vi "Periodic Tasks.vi"(8 "error in":errorcluster) -> ()   [LabVIEW 2012]
doc: "This VI runs in parallel to other tasks. It can contain as many user-defined periodic loops as you need. These can carry out PID or other sorts of timed response."
uses:
  <vilib>/Rock Robotics/SystemInterfaces/Utilities/FPGA_UtilitiesLED Source.ctl
  <vilib>/Rock Robotics/SystemInterfaces/Utilities/FPGA_UtilitiesLED State.ctl
  <vilib>/Rock Robotics/WPI/Solenoid/WPI_SolenoidValue.ctl
  Robot Global Data.vi
  <vilib>/Rock Robotics/WPI/Solenoid/WPI_SolenoidSetEnum.vi
  <vilib>/Rock Robotics/WPI/Compressor/WPI_CompressorGetSetRefNum.vi
panel:
  out "RawPot1":dbl
  out "RawGyro":dbl
  out "Pot1":dbl
  out "Gyro1":dbl
  out "PickupErrort":errorcluster
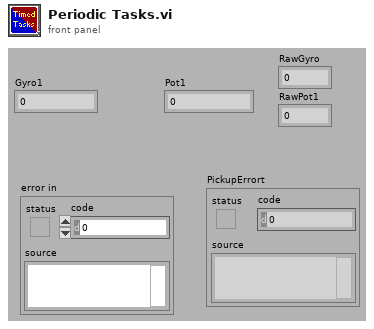
[diagram p1: front panel]
types:
  T1 = typedef "FPGA_UtilitiesLED State.ctl" = enum16{"Off", "On", "Toggle"}
  T2 = typedef "FPGA_UtilitiesLED Source.ctl" = enum16{"User LED", "FPGA LED"}
  T3 = typedef "WPI_MotorControlDeviceRef.ctl" = cluster{"DeviceStatus":errorcluster, "Type":enum16{"PWM", "CAN"}, "PWM":cluster{"Digital Module":T4, "PWM Channel":T5, "DeadBand":T6}, "CAN":cluster{"Device Number":u8, "Control Mode":T7, "Semaphore":T8, "Max Vout":dbl}, "Invert":bool, "TransformRef":T9, "InvTransformRef":T9}
  T4 = typedef "FPGA_TypedefDigitalModule.ctl" = enum16{"Digital Module 1", "Digital Module 2"}
  T5 = typedef "FPGA_DIOPWMChannel.ctl" = enum8{"PWM 1", "PWM 2", "PWM 3", "PWM 4", "PWM 5", "PWM 6", "PWM 7", "PWM 8", "PWM 9", "PWM 10", "Invalid"}
  T6 = typedef "WPI_PWMDeadband.ctl" = cluster{"Name":string, "maxPositivePwm":i32, "minPositivePwm":i32, "centerPwm":i32, "maxNegativePwm":i32, "minNegativePwm":i32, "angularRange":u16}
  T7 = typedef "WPI_CANJaguar_ControlMode.ctl" = enum8{"Percent VBus", "Current", "Speed", "Position", "Voltage"}
  T8 = typedef "Semaphore RefNum" = refnum<k1>
  T9 = typedef "WPI_PWMTransform_ConPane.ctl" = refnum<vi>
  T10 = typedef "WPI_SolenoidDevRef.ctl" = cluster{"DevStatus":errorcluster, "Solenoid Module":T11, "Forward Solenoid Channel":T12, "Reverse Solenoid Channel":T12}
  T11 = typedef "FPGA_TypedefSolenoidModule.ctl" = enum16{"Solenoid Module 1", "Solenoid Module 2"}
  T12 = typedef "WPI_SolenoidChannel.ctl" = enum8{"Solenoid 1", "Solenoid 2", "Solenoid 3", "Solenoid 4", "Solenoid 5", "Solenoid 6", "Solenoid 7", "Solenoid 8", "Invalid"}
  T13 = typedef "WPI_CompressorDevRef.ctl" = cluster{"DevStatus":errorcluster, "DigitalInputDevRef":T14, "RelayDevRef":T16}
  T14 = typedef "WPI_DigitalInputDevRef.ctl" = cluster{"DevStatus":errorcluster, "DIO Channel":T15, "Digital Module":T4}
  T15 = typedef "FPGA_DIOChannel.ctl" = enum8{"DIO 1", "DIO 2", "DIO 3", "DIO 4", "DIO 5", "DIO 6", "DIO 7", "DIO 8", "DIO 9", "DIO 10", "DIO 11", "DIO 12", "DIO 13", "DIO 14", "Invalid"}
  T16 = typedef "WPI_RelayDevRef.ctl" = cluster{"DevStatus":errorcluster, "Relay Channel":T17, "Digital Module":T4, "Relay Direction":T18}
  T17 = typedef "FPGA_DIORelayChannel.ctl" = enum8{"Relay 1", "Relay 2", "Relay 3", "Relay 4", "Relay 5", "Relay 6", "Relay 7", "Relay 8", "Invalid"}
  T18 = typedef "WPI_RelayDirection.ctl" = enum16{"Both directions", "Forward only", "Reverse only"}
  T19 = typedef "WPI_GyroDevRef.ctl" = cluster{"DevStatus":errorcluster, "Analog Module":T20, "Analog Channel":T21, "Offset":dbl, "Gain (VoltsPerDegree/Second)":dbl}
  T20 = typedef "FPGA_TypedefAnalogModule.ctl" = enum16{"Analog Module 1", "Analog Module 2"}
  T21 = typedef "FPGA_AIChannel.ctl" = enum8{"AI 1", "AI 2", "AI 3", "AI 4", "AI 5", "AI 6", "AI 7", "AI 8", "Invalid"}
  T22 = typedef "WPI_AnalogChannelDevRef.ctl" = cluster{"DevStatus":errorcluster, "Analog Module":T20, "Analog Channel":T21}
  T23 = enum16{"Reset", "Ready", "Down", "Capture", "Lift", "Swing", "Release"}
  T24 = typedef "WPI_SolenoidValue.ctl" = enum16{"Off", "On", "Forward", "Reverse"}
  T25 = cluster{"PizzaLow":dbl, "PizzaMid":dbl, "PizzaTop":dbl}
  T26 = cluster{"Shoot":bool, "Enable_Targeting":bool, "Shooter":dbl, "LeadScrew":dbl, "Feed":bool, "Pickup":bool}
  T27 = cluster{"Frisbee_Catch":bool, "Shooter_Ready":bool, "LeadScrewEnd":bool}
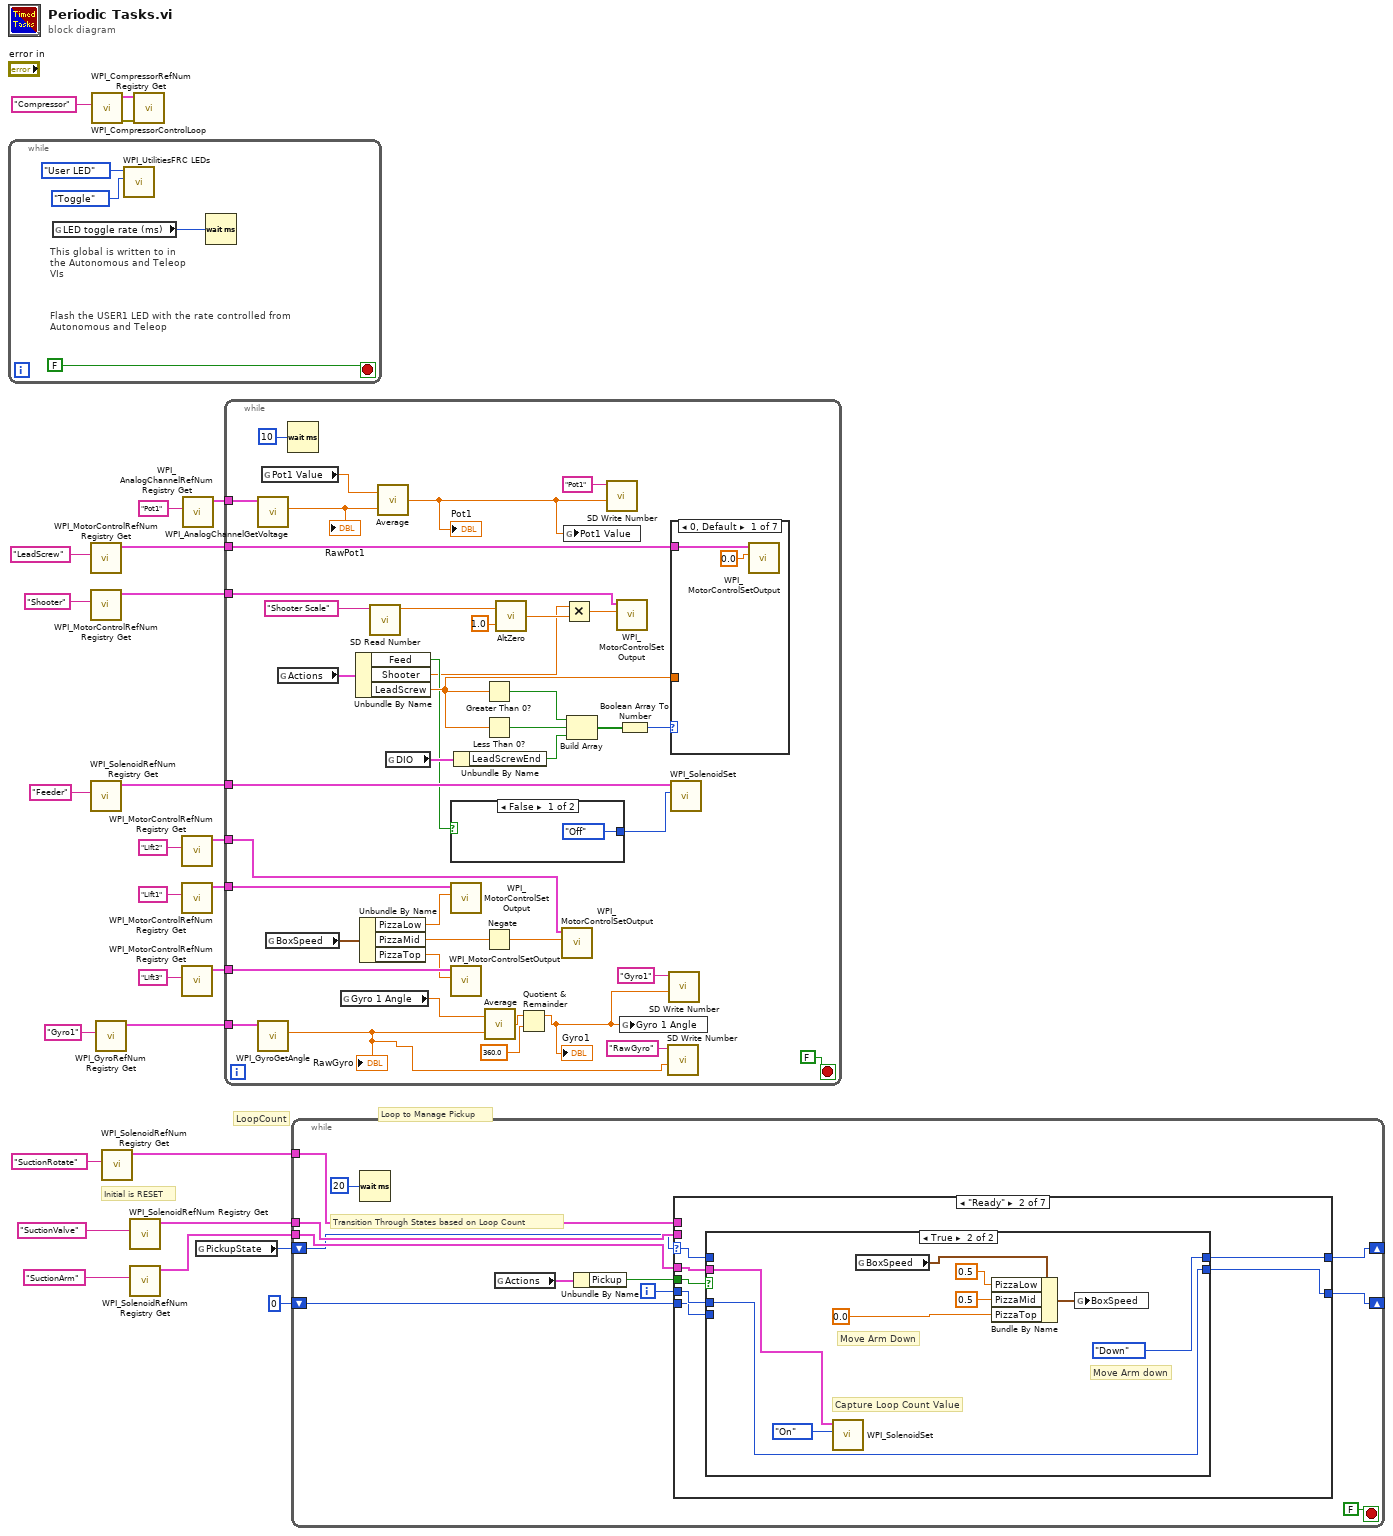
[diagram p0: block diagram]
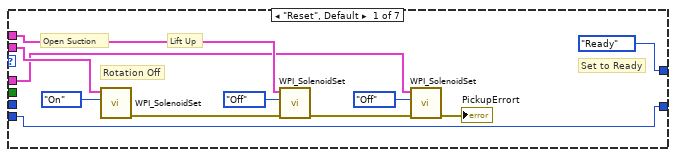
[diagram p2: hidden frame]
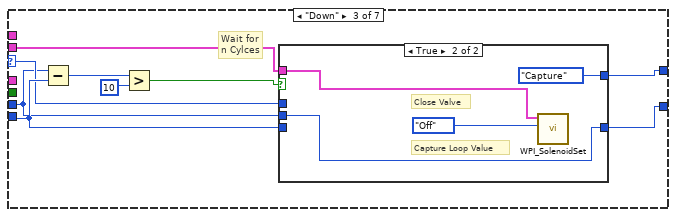
[diagram p4: hidden frame]
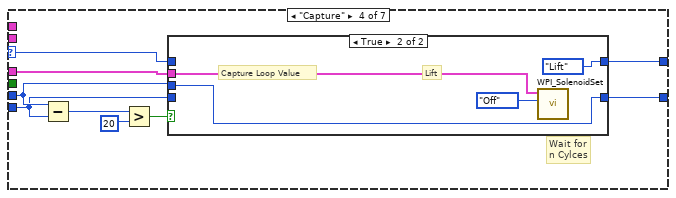
[diagram p6: hidden frame]
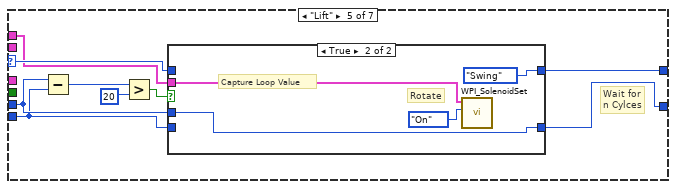
[diagram p8: hidden frame]
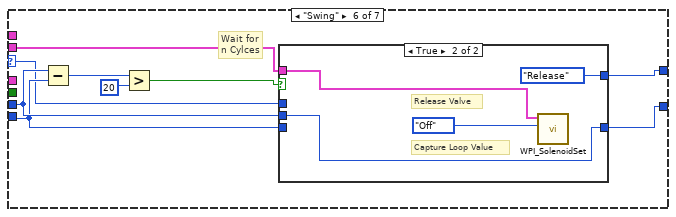
[diagram p10: hidden frame]
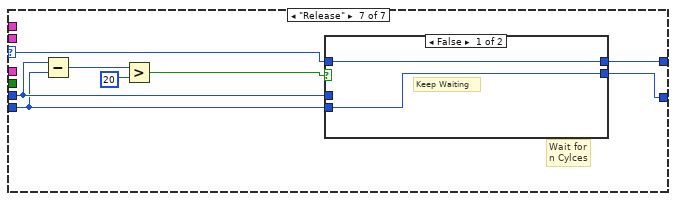
[diagram p12: hidden frame]
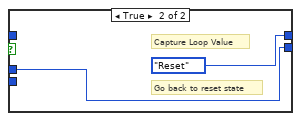
[diagram p13: hidden frame]
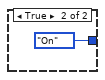
[diagram p14: hidden frame]
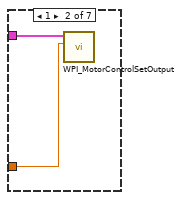
[diagram p15: hidden frame]
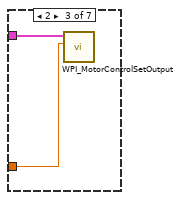
[diagram p16: hidden frame]
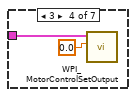
[diagram p17: hidden frame]
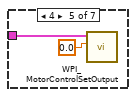
[diagram p18: hidden frame]
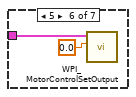
[diagram p19: hidden frame]
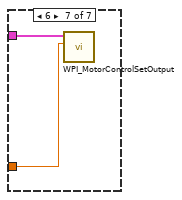
[diagram p20: hidden frame]
diagram:
  # "Initial is RESET"
  # "LoopCount"
  # "Loop to Manage Pickup"
  n1 = while {
    stop <- FALSE stop-if-true
    # "This global is written to in the Autonomous and Teleop VIs"
    # "Flash the USER1 LED with the rate controlled from Autonomous and Teleop"
    n2 = global read "Robot Global Data.vi" "LED toggle rate (ms)"() -> (w28:u32)
    n3 = call <vilib>:"WPI_UtilitiesFRC LEDs.vi"("State"=FPGA_UtilitiesLED_State."Toggle", "LED Type"=FPGA_UtilitiesLED_Source."User LED") -> ()  [unwired: 1 in, 9 out]
    n4 = Wait (ms)(milliseconds to wait=w28) -> ()  [unwired: 1 out]
  }
  n5 = call <vilib>:"WPI_MotorControlRefNum Registry Get.vi"("refnum name"="LeadScrew") -> ("MotorControlDevRef"=w23:T3)  [unwired: 9 in, 1 out]
  n6 = call <vilib>:"WPI_MotorControlRefNum Registry Get.vi"("refnum name"="Shooter") -> ("MotorControlDevRef"=w21:T3)  [unwired: 9 in, 1 out]
  n7 = call <vilib>:"WPI_SolenoidRefNum Registry Get.vi"("refnum name"="Feeder") -> ("SolenoidDevRef"=w20:T10)  [unwired: 9 in, 1 out]
  n8 = call <vilib>:"WPI_CompressorRefNum Registry Get.vi"("refnum name"="Compressor") -> ("error out"=w25:errorcluster, "CompressorDevRef"=w27:T13)  [unwired: 9 in]
  n9 = call <vilib>:"WPI_GyroRefNum Registry Get.vi"("refnum name"="Gyro1") -> ("GyroDevRef"=w3:T19)  [unwired: 9 in, 1 out]
  n10 = call <vilib>:"WPI_SolenoidRefNum Registry Get.vi"("refnum name"="SuctionRotate") -> ("SolenoidDevRef"=w13:T10)  [unwired: 9 in, 1 out]
  n11 = call <vilib>:"WPI_SolenoidRefNum Registry Get.vi"("refnum name"="SuctionValve") -> ("SolenoidDevRef"=w15:T10)  [unwired: 9 in, 1 out]
  n12 = call <vilib>:"WPI_SolenoidRefNum Registry Get.vi"("refnum name"="SuctionArm") -> ("SolenoidDevRef"=w14:T10)  [unwired: 9 in, 1 out]
  n13 = call <vilib>:"WPI_CompressorControlLoop.vi"("error in (no error)"=w25, "CompressorDevRef"=w27) -> ()  [unwired: 10 in]
  n14 = call <vilib>:"WPI_MotorControlRefNum Registry Get.vi"("refnum name"="Lift2") -> ("MotorControlDevRef"=w5:T3)  [unwired: 9 in, 1 out]
  n15 = call <vilib>:"WPI_MotorControlRefNum Registry Get.vi"("refnum name"="Lift1") -> ("MotorControlDevRef"=w7:T3)  [unwired: 9 in, 1 out]
  n16 = call <vilib>:"WPI_MotorControlRefNum Registry Get.vi"("refnum name"="Lift3") -> ("MotorControlDevRef"=w6:T3)  [unwired: 9 in, 1 out]
  n17 = call <vilib>:"WPI_AnalogChannelRefNum Registry Get.vi"("refnum name"="Pot1") -> ("AIDeviceRef"=w1:T22)  [unwired: 9 in, 1 out]
  n18 = global read "Robot Global Data.vi" "PickupState"() -> (w12:T23)
  n19 = while {
    tunnel: w23 -> [w66]
    tunnel: w21 -> [w65]
    tunnel: w20 -> [w61]
    tunnel: w7 -> [w57]
    tunnel: w6 -> [w56]
    tunnel: w5 -> [w55]
    tunnel: w3 -> [w50]
    tunnel: w1 -> [w42]
    stop <- FALSE stop-if-true
    n20 = call <vilib>:"WPI_AnalogChannelGetVoltage.vi"("AIDeviceRef"=w42) -> ("Voltage"=w39:dbl)  [unwired: 8 in, 2 out]
    "RawPot1" <- w39
    n21 = call <vilib>:"WPI_GyroGetAngle.vi"("GyroDevRef"=w50) -> ("Angle"=w33:dbl)  [unwired: 7 in, 3 out]
    "RawGyro" <- w33
    n22 = global read "Robot Global Data.vi" "Pot1 Value"() -> (w40:dbl)
    n23 = global read "Robot Global Data.vi" "BoxSpeed"() -> (w58:T25)
    n24 = global read "Robot Global Data.vi" "Actions"() -> (w64:T26)
    n25 = Wait (ms)(milliseconds to wait=u32 10) -> ()  [unwired: 1 out]
    n26 = global read "Robot Global Data.vi" "Gyro 1 Angle"() -> (w41:dbl)
    n27 = Unbundle By Name(w64) -> ("Feed"=w59:bool, "Shooter"=w44:dbl, "LeadScrew"=w60:dbl)
    n28 = Unbundle By Name(w58) -> ("PizzaLow"=w54:dbl, "PizzaMid"=w52:dbl, "PizzaTop"=w51:dbl)
    n29 = call <vilib>:"SD Read Number.vi"("Name"="Shooter Scale") -> ("Numeric"=w46:dbl)  [unwired: 8 in, 2 out]
    n30 = call "Average.vi"("z"=w39, "x"=w40) -> ("y"=w38:dbl)
    "Pot1" <- w38
    n31 = global read "Robot Global Data.vi" "DIO"() -> (w63:T27)
    n32 = case shown="False" w59 {
      tunnel: [WPI_SolenoidValue."Off" ("Value") WPI_SolenoidValue."On" ("Value")] -> w62
      frame False {
      }
      frame True {
      }
    }
    n33 = call <vilib>:"WPI_MotorControlSetOutput.vi"("Output"=w54, "MotorControlDevRef"=w57) -> ()  [unwired: 7 in, 3 out]
    n34 = call <vilib>:"WPI_MotorControlSetOutput.vi"("Output"=w51, "MotorControlDevRef"=w56) -> ()  [unwired: 7 in, 3 out]
    n35 = Unbundle By Name(w63) -> ("LeadScrewEnd"=w67:bool)
    n36 = Greater Than 0?(x=w60) -> (x > 0?=w70:bool)
    n37 = Less Than 0?(x=w60) -> (x < 0?=w71:bool)
    n38 = Negate(x=w52) -> (-x=w53:dbl)
    n39 = call "Average.vi"("z"=w33, "x"=w41) -> ("y"=w36:dbl)
    n40 = call "AltZero.vi"("z"=1.0, "x"=w46) -> ("y"=w47:dbl)
    n41 = Quotient & Remainder(x=w36, y=360.0) -> (x-y*floor(x/y)=w35:dbl)  [unwired: 1 out]
    "Gyro1" <- w35
    n42 = call <vilib>:"WPI_MotorControlSetOutput.vi"("Output"=w53, "MotorControlDevRef"=w55) -> ()  [unwired: 7 in, 3 out]
    n43 = global write "Robot Global Data.vi" "Pot1 Value"(w38) -> ()
    n44 = Multiply(x=w44, y=w47) -> (x*y=w43:dbl)
    n45 = Build Array(w70, w71, w67) -> (w69:bool[])
    n46 = call <vilib>:"SD Write Number.vi"("Numeric"=w38, "Name"="Pot1") -> ()  [unwired: 8 in, 2 out]
    n47 = call <vilib>:"WPI_MotorControlSetOutput.vi"("Output"=w43, "MotorControlDevRef"=w65) -> ()  [unwired: 7 in, 3 out]
    n48 = Boolean Array To Number(Boolean array=w69) -> (number=w68:u32)
    n49 = global write "Robot Global Data.vi" "Gyro 1 Angle"(w35) -> ()
    n50 = call <vilib>:"SD Write Number.vi"("Numeric"=w33, "Name"="RawGyro") -> ()  [unwired: 8 in, 2 out]
    n51 = call <vilib>:"SD Write Number.vi"("Numeric"=w35, "Name"="Gyro1") -> ()  [unwired: 8 in, 2 out]
    n52 = case shown="0, Default" w68 {
      tunnel: w60 -> [_ w79 w81 _ _ _ w88]
      tunnel: w66 -> [w76 w78 w80 w83 w85 w87 w89]
      frame 0, Default {
        n53 = call <vilib>:"WPI_MotorControlSetOutput.vi"("Output"=0.0, "MotorControlDevRef"=w76) -> ()  [unwired: 7 in, 3 out]
      }
      frame 1 {
        n54 = call <vilib>:"WPI_MotorControlSetOutput.vi"("Output"=w79, "MotorControlDevRef"=w78) -> ()  [unwired: 7 in, 3 out]
      }
      frame 2 {
        n55 = call <vilib>:"WPI_MotorControlSetOutput.vi"("Output"=w81, "MotorControlDevRef"=w80) -> ()  [unwired: 7 in, 3 out]
      }
      frame 3 {
        n56 = call <vilib>:"WPI_MotorControlSetOutput.vi"("Output"=0.0, "MotorControlDevRef"=w83) -> ()  [unwired: 7 in, 3 out]
      }
      frame 4 {
        n57 = call <vilib>:"WPI_MotorControlSetOutput.vi"("Output"=0.0, "MotorControlDevRef"=w85) -> ()  [unwired: 7 in, 3 out]
      }
      frame 5 {
        n58 = call <vilib>:"WPI_MotorControlSetOutput.vi"("Output"=0.0, "MotorControlDevRef"=w87) -> ()  [unwired: 7 in, 3 out]
      }
      frame 6 {
        n59 = call <vilib>:"WPI_MotorControlSetOutput.vi"("Output"=w88, "MotorControlDevRef"=w89) -> ()  [unwired: 7 in, 3 out]
      }
    }
    n60 = call-poly <vilib>:"WPI_SolenoidSet.vi"("Value"=w62, "SolenoidDevRef"=w61) -> ()  [unwired: 8 in, 2 out]
  }
  n61 = while {
    tunnel: w15 -> [w99]
    tunnel: w14 -> [w98]
    tunnel: w13 -> [w97]
    shift-right: [w96] -> _
    shift-left: w12 -> [w95]
    shift-right: [w90] -> _
    shift-left: 0 -> [w91]
    i -> [w92]
    stop <- FALSE stop-if-true
    # "Transition Through States based on Loop Count"
    n62 = Wait (ms)(milliseconds to wait=u32 20) -> ()  [unwired: 1 out]
    n63 = global read "Robot Global Data.vi" "Actions"() -> (w94:T26)
    n64 = Unbundle By Name(w94) -> ("Pickup"=w93:bool)
    n65 = case shown="\"Ready\"" w95 {
      selector: w95 -> [_ w113 w134 w151 w162 w177 w193]
      tunnel: w99 -> [w112 _ w131 _ _ w176 _]
      tunnel: w98 -> [w103 w117 _ w148 _ _ _]
      tunnel: w97 -> [w104 _ _ _ w161 _ _]
      tunnel: [T23."Ready" ("PickupState") w118 w133 w147 w163 w181 w192] -> w96
      tunnel: w93 -> [_ w119 _ _ _ _ _]
      tunnel: w92 -> [_ w116 w132 w150 w166 w179 w195]
      tunnel: w91 -> [w105 w114 w136 w149 w165 w178 w194]
      tunnel: [w105 w115 w135 w146 w164 w180 w191] -> w90
      frame "Reset", Default {
        # "Set to Ready"
        # "Rotation Off"
        # "Lift Up"
        # "Open Suction"
        n66 = call-poly <vilib>:"WPI_SolenoidSet.vi"("Value"=WPI_SolenoidValue."On", "SolenoidDevRef"=w112) -> ("error out"=w109:errorcluster)  [unwired: 8 in, 1 out]
        n67 = call-poly <vilib>:"WPI_SolenoidSet.vi"("error in (no error)"=w109, "Value"=WPI_SolenoidValue."Off", "SolenoidDevRef"=w104) -> ("error out"=w102:errorcluster)  [unwired: 7 in, 1 out]
        n68 = call-poly <vilib>:"WPI_SolenoidSet.vi"("error in (no error)"=w102, "Value"=WPI_SolenoidValue."Off", "SolenoidDevRef"=w103) -> ("error out"=→"PickupErrort":errorcluster)  [unwired: 7 in, 1 out]
      }
      frame "Ready" {
        n69 = case shown="True" w119 {
          tunnel: [w120 T23."Down" ("PickupState")] -> w118
          tunnel: w117 -> [_ w129]
          tunnel: w116 -> [_ w127]
          tunnel: [w121 w127] -> w115
          tunnel: w114 -> [w121 _]
          tunnel: w113 -> [w120 _]
          frame False {
            # "Pass state\nand Loop\nCount"
          }
          frame True {
            # "Move Arm down"
            # "Capture Loop Count Value"
            # "Move Arm Down"
            n70 = call-poly <vilib>:"WPI_SolenoidSet.vi"("Value"=WPI_SolenoidValue."On", "SolenoidDevRef"=w129) -> ()  [unwired: 8 in, 2 out]
            n71 = global read "Robot Global Data.vi" "BoxSpeed"() -> (w126:T25)
            n72 = Bundle By Name(cluster=w126, "PizzaLow"=0.5, "PizzaMid"=0.5, "PizzaTop"=0.0) -> (w122:T25)
            n73 = global write "Robot Global Data.vi" "BoxSpeed"(w122) -> ()
          }
        }
      }
      frame "Down" {
        # "Wait for\nn Cylces"
        n74 = Subtract(x=w132, y=w136) -> (x-y=w139:i32)
        n75 = Greater?(x=w139, y=10) -> (0:w137:bool)
        n76 = case shown="True" w137 {
          tunnel: w136 -> [w141 _]
          tunnel: [w141 w145] -> w135
          tunnel: w134 -> [w140 _]
          tunnel: [w140 T23."Capture" ("PickupState")] -> w133
          tunnel: w132 -> [_ w145]
          tunnel: w131 -> [_ w144]
          frame False {
            # "Keep Waiting"
          }
          frame True {
            # "Capture Loop Value"
            # "Close Valve"
            n77 = call-poly <vilib>:"WPI_SolenoidSet.vi"("Value"=WPI_SolenoidValue."Off", "SolenoidDevRef"=w144) -> ()  [unwired: 8 in, 2 out]
          }
        }
      }
      frame "Capture" {
        # "Wait for\nn Cylces"
        n78 = Subtract(x=w150, y=w149) -> (x-y=w154:i32)
        n79 = Greater?(x=w154, y=20) -> (0:w152:bool)
        n80 = case shown="True" w152 {
          tunnel: w149 -> [w156 _]
          tunnel: [w156 w160] -> w146
          tunnel: w151 -> [w155 _]
          tunnel: [w155 T23."Lift" ("PickupState")] -> w147
          tunnel: w150 -> [_ w160]
          tunnel: w148 -> [_ w159]
          frame False {
            # "Keep Waiting"
          }
          frame True {
            # "Capture Loop Value"
            # "Lift"
            n81 = call-poly <vilib>:"WPI_SolenoidSet.vi"("Value"=WPI_SolenoidValue."Off", "SolenoidDevRef"=w159) -> ()  [unwired: 8 in, 2 out]
          }
        }
      }
      frame "Lift" {
        # "Wait for\nn Cylces"
        n82 = Subtract(x=w166, y=w165) -> (x-y=w169:i32)
        n83 = Greater?(x=w169, y=20) -> (0:w167:bool)
        n84 = case shown="True" w167 {
          tunnel: w165 -> [w171 _]
          tunnel: [w171 w175] -> w164
          tunnel: w162 -> [w170 _]
          tunnel: [w170 T23."Swing" ("PickupState")] -> w163
          tunnel: w166 -> [_ w175]
          tunnel: w161 -> [_ w174]
          frame False {
            # "Keep Waiting"
          }
          frame True {
            # "Capture Loop Value"
            # "Rotate"
            n85 = call-poly <vilib>:"WPI_SolenoidSet.vi"("Value"=WPI_SolenoidValue."On", "SolenoidDevRef"=w174) -> ()  [unwired: 8 in, 2 out]
          }
        }
      }
      frame "Swing" {
        # "Wait for\nn Cylces"
        n86 = Subtract(x=w179, y=w178) -> (x-y=w184:i32)
        n87 = Greater?(x=w184, y=20) -> (0:w182:bool)
        n88 = case shown="True" w182 {
          tunnel: w178 -> [w186 _]
          tunnel: [w186 w190] -> w180
          tunnel: w177 -> [w185 _]
          tunnel: [w185 T23."Release" ("PickupState")] -> w181
          tunnel: w179 -> [_ w190]
          tunnel: w176 -> [_ w189]
          frame False {
            # "Keep Waiting"
          }
          frame True {
            # "Capture Loop Value"
            # "Release Valve"
            n89 = call-poly <vilib>:"WPI_SolenoidSet.vi"("Value"=WPI_SolenoidValue."Off", "SolenoidDevRef"=w189) -> ()  [unwired: 8 in, 2 out]
          }
        }
      }
      frame "Release" {
        # "Wait for\nn Cylces"
        n90 = Subtract(x=w195, y=w194) -> (x-y=w198:i32)
        n91 = Greater?(x=w198, y=20) -> (0:w196:bool)
        n92 = case shown="False" w196 {
          tunnel: w194 -> [w200 _]
          tunnel: [w200 w202] -> w191
          tunnel: w193 -> [w199 _]
          tunnel: [w199 T23."Reset" ("PickupState")] -> w192
          tunnel: w195 -> [_ w202]
          frame False {
            # "Keep Waiting"
          }
          frame True {
            # "Go back to reset state"
            # "Capture Loop Value"
          }
        }
      }
    }
  }
